vi "SPARK Get Status 1.vi"(8 "error in (no error)":errorcluster, 11 "MotorControlDevRef":T4) -> (0 "error out":errorcluster, 2 "Status 1":T1, 3 "MotorControlDevRef":T4)   [LabVIEW 2023]
uses:
  Typedef/Spark MAX Variant Data.ctl
  Typedef/SPARK Model.ctl
  Typedef/SPARK CAN Arb ID.ctl
  Typedef/SPARK Faults.ctl
  Typedef/SPARK Warnings.ctl
  Typedef/SPARK Status 1 Frame.ctl
  Typedef/SPARK Periodic Status.ctl
  <vilib>/Rock Robotics/SystemInterfaces/DIO/FPGA_DIOPWMChannel.ctl
  <vilib>/Rock Robotics/WPI/PWM/WPI_PWMDeadband.ctl
  <vilib>/Rock Robotics/WPI/MotorControl/WPI_MotorControlType.ctl
  <vilib>/Rock Robotics/SystemInterfaces/DIO/FPGA_DIOChannel.ctl
  <vilib>/Rock Robotics/WPI/MotorControl/WPI_MotorControlDeviceRef.ctl
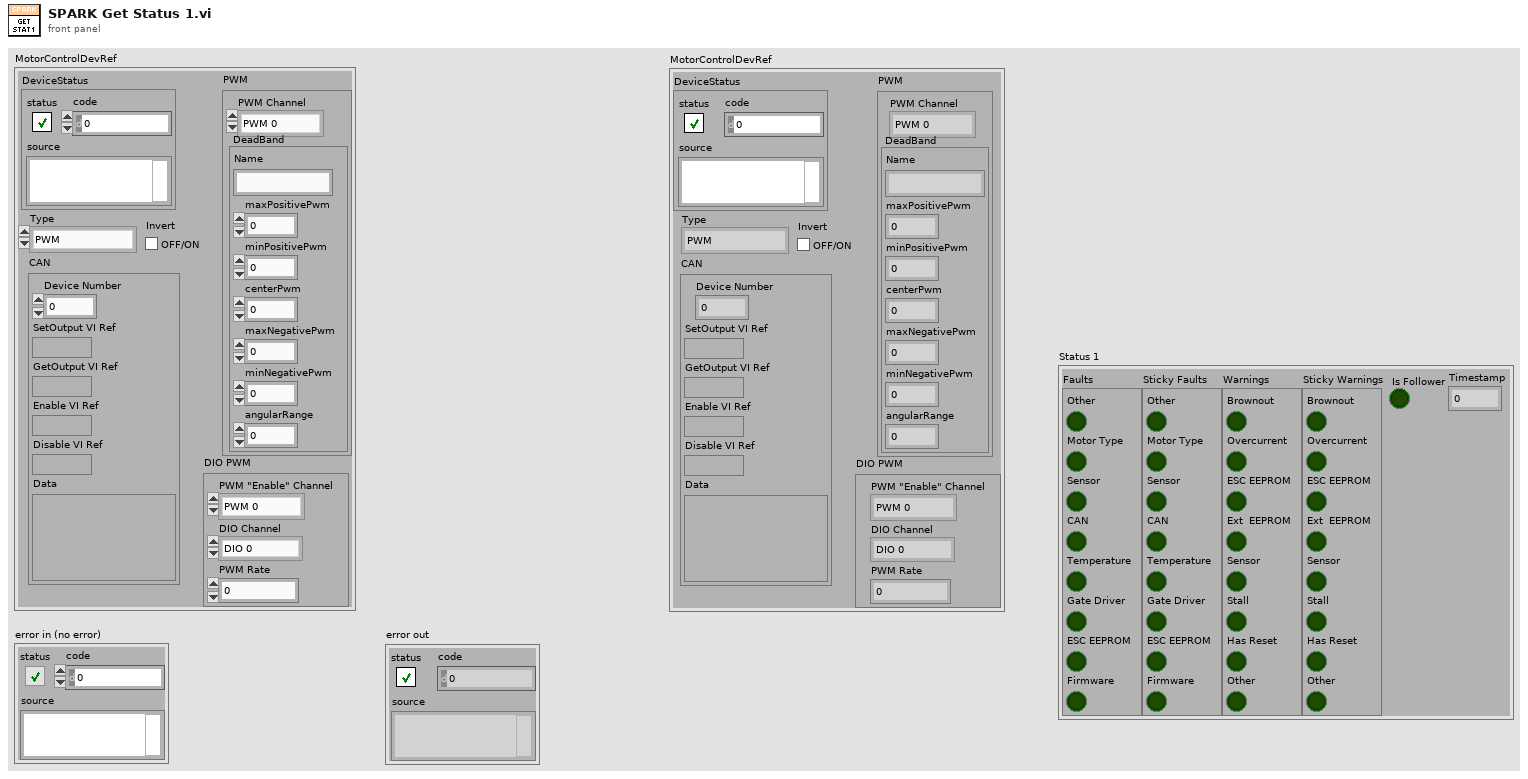
[diagram p1: front panel]
types:
  T1 = typedef "SPARK Status 1 Frame.ctl" = cluster{"Faults":T2, "Sticky Faults":T2, "Warnings":T3, "Sticky Warnings":T3, "Is Follower":bool, "Timestamp":u32}
  T2 = typedef "SPARK Faults.ctl" = cluster{"Other":bool, "Motor Type":bool, "Sensor":bool, "CAN":bool, "Temperature":bool, "Gate Driver":bool, "ESC EEPROM":bool, "Firmware":bool}
  T3 = typedef "SPARK Warnings.ctl" = cluster{"Brownout":bool, "Overcurrent":bool, "ESC EEPROM":bool, "Ext  EEPROM":bool, "Sensor":bool, "Stall":bool, "Has Reset":bool, "Other":bool}
  T4 = typedef "WPI_MotorControlDeviceRef.ctl" = cluster{"DeviceStatus":errorcluster, "Type":T5, "PWM":cluster{"PWM Channel":T6, "DeadBand":T7}, "CAN":cluster{"Device Number":u8, "SetOutput VI Ref":variant, "GetOutput VI Ref":variant, "Enable VI Ref":variant, "Disable VI Ref":variant, "Data":variant}, "Invert":bool, "DIO PWM":cluster{"PWM \"Enable\" Channel":T6, "DIOChannel":T8, "PWM Rate":dbl}}
  T5 = typedef "WPI_MotorControlType.ctl" = enum16{"PWM", "CAN", "DIO PWM"}
  T6 = typedef "FPGA_DIOPWMChannel.ctl" = enum8{"PWM 0", "PWM 1", "PWM 2", "PWM 3", "PWM 4", "PWM 5", "PWM 6", "PWM 7", "PWM 8", "PWM 9", "PWM MXP 0", "PWM MXP 1", "PWM MXP 2", "PWM MXP 3", "PWM MXP 4", "PWM MXP 5", "PWM MXP 6", "PWM MXP 7", "PWM MXP 8", "PWM MXP 9", "Invalid"}
  T7 = typedef "WPI_PWMDeadband.ctl" = cluster{"Name":string, "maxPositivePwm":i32, "minPositivePwm":i32, "centerPwm":i32, "maxNegativePwm":i32, "minNegativePwm":i32, "angularRange":u16}
  T8 = typedef "FPGA_DIOChannel.ctl" = enum8{"DIO 0", "DIO 1", "DIO 2", "DIO 3", "DIO 4", "DIO 5", "DIO 6", "DIO 7", "DIO 8", "DIO 9", "DIO MXP 0", "DIO MXP 1", "DIO MXP 2", "DIO MXP 3", "DIO MXP 4", "DIO MXP 5", "DIO MXP 6", "DIO MXP 7", "DIO MXP 8", "DIO MXP 9", "DIO MXP 10", "DIO MXP 11", "DIO MXP 12", "DIO MXP 13", "DIO MXP 14", "DIO MXP 15", "SPI Port CS1", "SPI Port CS2", "SPI Port CS3", "SPI Port MISO", "SPI Port MOSI", "Invalid"}
  T9 = typedef "SPARK Periodic Status.ctl" = enum16{"Periodic Status 0", "Periodic Status 1", "Periodic Status 2", "Periodic Status 3", "Periodic Status 4", "Periodic Status 5", "Periodic Status 6", "Periodic Status 7"}
  T10 = typedef "SPARK CAN Arb ID.ctl" = u32
  T11 = typedef "Spark MAX Variant Data.ctl" = cluster{"Ext ID":u32, "CAN Timeout":u32, "Inverted No WPILib":bool, "Has Configured Limit Sw":bool, "Has Configured Alt Encoder":bool, "SPARK Model":T12, "CAN Max Retries":u32, "CAN Timeout (ms)":u32, "Status 0 Period (ms)":u32, "Status 1 Period (ms)":u32, "Status 2 Period (ms)":u32, "Status 3 Period (ms)":u32, "Status 4 Period (ms)":u32, "Status 5 Period (ms)":u32, "Status 6 Period (ms)":u32, "Status 7 Period (ms)":u32, "Status Frame Timeout (ms)":u32}
  T12 = typedef "SPARK Model.ctl" = enum16{"SPARK MAX", "SPARK Flex", "Unknown"}
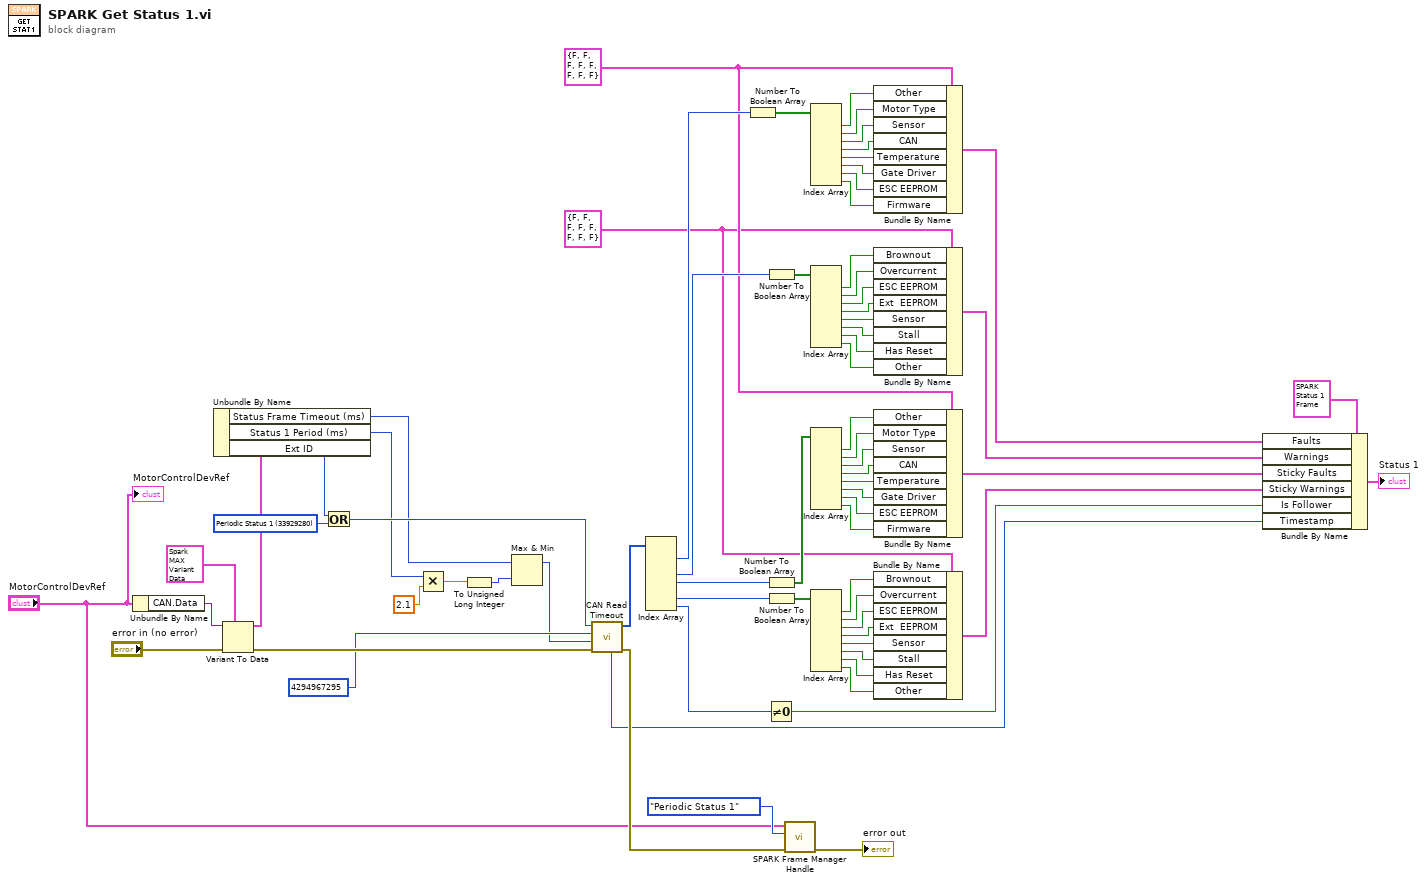
[diagram p0: block diagram]
diagram:
  w13 = T3 {"Brownout"=FALSE, "Overcurrent"=FALSE, "ESC EEPROM"=FALSE, "Ext  EEPROM"=FALSE, "Sensor"=FALSE, "Stall"=FALSE, "Has Reset"=FALSE, "Other"=FALSE} ("Warnings")
  w14 = T2 {"Other"=FALSE, "Motor Type"=FALSE, "Sensor"=FALSE, "CAN"=FALSE, "Temperature"=FALSE, "Gate Driver"=FALSE, "ESC EEPROM"=FALSE, "Firmware"=FALSE} ("Faults")
  w66 = T10 33929280 items=["Broadcast Disable"=0, "Broadcast System Halt"=64, "Broadcast System Reset"=128, "Broadcast Device Assign"=192, "Broadcast Heartbeat"=320, "Broadcast Firmware Version"=512, "Broadcast Enumerate"=576, "Broadcast System Resume"=640, "Velocity Setpoint"=33882112, "Duty Cycle Setpoint"=33882240, "Smart Velocity Setpoint"=33882304, "Position Setpoint"=33882368, "Voltage Setpoint"=33882432, "Current Setpoint"=33882496, "Smart Motion Setpoint"=33882560, "MAXMotion Position Setpoint"=33882624, "MAXMotion Velocity Setpoint"=33882688, "Periodic Status 0"=33929216, "Periodic Status 1"=33929280, "Periodic Status 2"=33929344, "Periodic Status 3"=33929408, "Periodic Status 4"=33929472, "Periodic Status 5"=33929536, "Periodic Status 6"=33929600, "Periodic Status 7"=33929664, "DRV Status"=33888896, "Clear Faults"=33889152, "Set Config Parameter"=33889280, "Get Config Parameter"=33889344, "Config Burn Flash"=33889408, "Set Follower Mode"=33889472, "Config Factory Defaults"=33889536, "Config Factory Reset"=33889600, "Nack"=33890304, "Ack"=33890368, "Broadcast (not a command)"=33891328, "Heartbeat"=33891456, "Sync"=33891520, "IDQuery"=33891584, "IDAssign"=33891648, "Firmware Version"=33891840, "REV Enumerate"=33891904, "Legacy/USB Heartbeat"=33891968, "roboRIO Lock"=33892032, "SWDL Data"=33892096, "SWDL Checksum"=33892160, "SWDL Retransmit"=33892224, "Telemetry Update Mechanical Position Enoder Port"=33892352, "Telemetry Update I Accum"=33892480, "Telemtry Update Mechanical Position Alt Encoder"=33892608, "Telemetry Update Mechanical Position Analog"=33892544, "Non-roboRIO Broadcast (not a command)"=33893376, "non-RIO Lock"=33893440, "non-RIO Heartbeat"=33893504] ("SPARK Arb ID")
  n1 = Unbundle By Name("MotorControlDevRef") -> ("CAN.Data"=w68:variant)
  n2 = Variant To Data(error in="error in (no error)", type=T11 {"Ext ID"=0, "CAN Timeout"=0, "Inverted No WPILib"=FALSE, "Has Configured Limit Sw"=FALSE, "Has Configured Alt Encoder"=FALSE, "SPARK Model"=enum."Unknown", "CAN Max Retries"=5, "CAN Timeout (ms)"=20, "Status 0 Period (ms)"=10, "Status 1 Period (ms)"=250, "Status 2 Period (ms)"=20, "Status 3 Period (ms)"=20, "Status 4 Period (ms)"=20, "Status 5 Period (ms)"=20, "Status 6 Period (ms)"=20, "Status 7 Period (ms)"=20, "Status Frame Timeout (ms)"=500} ("SPARK TNG Device Ref"), Variant=w68) -> (data=w70:T11, error out=w64:errorcluster)
  n3 = Unbundle By Name(w70) -> ("Status Frame Timeout (ms)"=w3:u32, "Status 1 Period (ms)"=w2:u32, "Ext ID"=w67:u32)
  n4 = Or(x=w67, y=w66) -> (x .or. y?=w65:T10)
  n5 = Multiply(x=w2, y=2.1) -> (x*y=w5:dbl)
  n6 = To Unsigned Long Integer(number=w5) -> (unsigned 32bit integer=w4:u32)
  n7 = Max & Min(x=w3, y=w4) -> (max(x,y)=w1:u32)  [unwired: 1 out]
  n8 = call "CAN Read Timeout.vi"("error in (no error)"=w64, "Timeout (ms)"=w1, "Message ID Mask"=u32 4294967295, "Message ID"=w65) -> ("error out"=w11:errorcluster, "data"=w61:u8[], "timestamp"=w7:u32)  [unwired: 5 in]
  n9 = Index Array(array=w61) -> (element #1=w60:u8, element #3=w40:u8, element #4=w29:u8, element #6=w18:u8, element #7=w16:u8)  [unwired: 7 in, 2 out]
  n10 = Number To Boolean Array(number=w60) -> (Boolean array=w59:bool[])
  n11 = Not Equal To 0?(x=w16) -> (x != 0?=w15:bool)
  n12 = Number To Boolean Array(number=w40) -> (Boolean array=w42:bool[])
  n13 = Number To Boolean Array(number=w29) -> (Boolean array=w30:bool[])
  n14 = Number To Boolean Array(number=w18) -> (Boolean array=w26:bool[])
  n15 = call "SPARK Frame Manager Handle.vi"("error in (no error)"=w11, "Periodic Status"=SPARK_Periodic_Status."Periodic Status 1", "MotorControlDeviceRef"="MotorControlDevRef") -> ("error out"=→"error out":errorcluster)  [unwired: 8 in]
  n16 = Index Array(array=w59) -> (element #1=w58:bool, element #2=w57:bool, element #3=w56:bool, element #4=w55:bool, element #5=w54:bool, element #6=w53:bool, element #7=w52:bool, element #8=w51:bool)  [unwired: 8 in]
  n17 = Index Array(array=w42) -> (element #1=w41:bool, element #2=w43:bool, element #3=w44:bool, element #4=w45:bool, element #5=w46:bool, element #6=w47:bool, element #7=w48:bool, element #8=w49:bool)  [unwired: 8 in]
  n18 = Index Array(array=w30) -> (element #1=w31:bool, element #2=w32:bool, element #3=w33:bool, element #4=w34:bool, element #5=w35:bool, element #6=w36:bool, element #7=w37:bool, element #8=w38:bool)  [unwired: 8 in]
  n19 = Index Array(array=w26) -> (element #1=w27:bool, element #2=w25:bool, element #3=w24:bool, element #4=w23:bool, element #5=w22:bool, element #6=w21:bool, element #7=w20:bool, element #8=w19:bool)  [unwired: 8 in]
  n20 = Bundle By Name(cluster=w14, "Other"=w58, "Motor Type"=w57, "Sensor"=w56, "CAN"=w55, "Temperature"=w54, "Gate Driver"=w53, "ESC EEPROM"=w52, "Firmware"=w51) -> (w50:T2)
  n21 = Bundle By Name(cluster=w13, "Brownout"=w41, "Overcurrent"=w43, "ESC EEPROM"=w44, "Ext  EEPROM"=w45, "Sensor"=w46, "Stall"=w47, "Has Reset"=w48, "Other"=w49) -> (w39:T3)
  n22 = Bundle By Name(cluster=w14, "Other"=w31, "Motor Type"=w32, "Sensor"=w33, "CAN"=w34, "Temperature"=w35, "Gate Driver"=w36, "ESC EEPROM"=w37, "Firmware"=w38) -> (w28:T2)
  n23 = Bundle By Name(cluster=w13, "Brownout"=w27, "Overcurrent"=w25, "ESC EEPROM"=w24, "Ext  EEPROM"=w23, "Sensor"=w22, "Stall"=w21, "Has Reset"=w20, "Other"=w19) -> (w17:T3)
  n24 = Bundle By Name(cluster=T1 {"Faults"={"Other"=FALSE, "Motor Type"=FALSE, "Sensor"=FALSE, "CAN"=FALSE, "Temperature"=FALSE, "Gate Driver"=FALSE, "ESC EEPROM"=FALSE, "Firmware"=FALSE}, "Sticky Faults"={"Other"=FALSE, "Motor Type"=FALSE, "Sensor"=FALSE, "CAN"=FALSE, "Temperature"=FALSE, "Gate Driver"=FALSE, "ESC EEPROM"=FALSE, "Firmware"=FALSE}, "Warnings"={"Brownout"=FALSE, "Overcurrent"=FALSE, "ESC EEPROM"=FALSE, "Ext  EEPROM"=FALSE, "Sensor"=FALSE, "Stall"=FALSE, "Has Reset"=FALSE, "Other"=FALSE}, "Sticky Warnings"={"Brownout"=FALSE, "Overcurrent"=FALSE, "ESC EEPROM"=FALSE, "Ext  EEPROM"=FALSE, "Sensor"=FALSE, "Stall"=FALSE, "Has Reset"=FALSE, "Other"=FALSE}, "Is Follower"=FALSE, "Timestamp"=0} ("SPARK Status 1"), "Faults"=w50, "Warnings"=w39, "Sticky Faults"=w28, "Sticky Warnings"=w17, "Is Follower"=w15, "Timestamp"=w7) -> (→"Status 1":T1)
  "MotorControlDevRef" <- "MotorControlDevRef"
